vi "Convert_command_string_to_Enum.vi"(5 "Command field in":string, 11 "error in (no error)":errorcluster) -> (6 "mmW_instrument_commands":T1, 10 "Found in Enum?":bool, 15 "error out":errorcluster)   [LabVIEW 2019, in "mmW_commands.lvlib"]
uses:
  mmW_commands.lvlib
  TypeDefs/commands.ctl
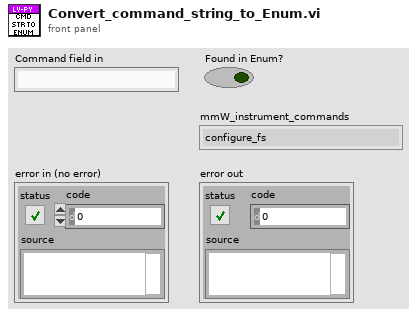
[diagram p1: front panel]
types:
  T1 = typedef "mmW_commands.lvlib/commands.ctl" = enum16{"configure_fs", "configure_rf", "configure_trigger", "equalization_enable", "equalization_start", "lo_sync_enable", "equalization_stop", "get_instrument_status", "get_versions", "initialize_hw", "pop_rx", "set_log_level", "Shutdown", "start", "start_instrument_app", "stop", "transceive", "trigger_burst", "trigger_sync_enable", "Write TX", "resp_generic", "resp_waveform"}
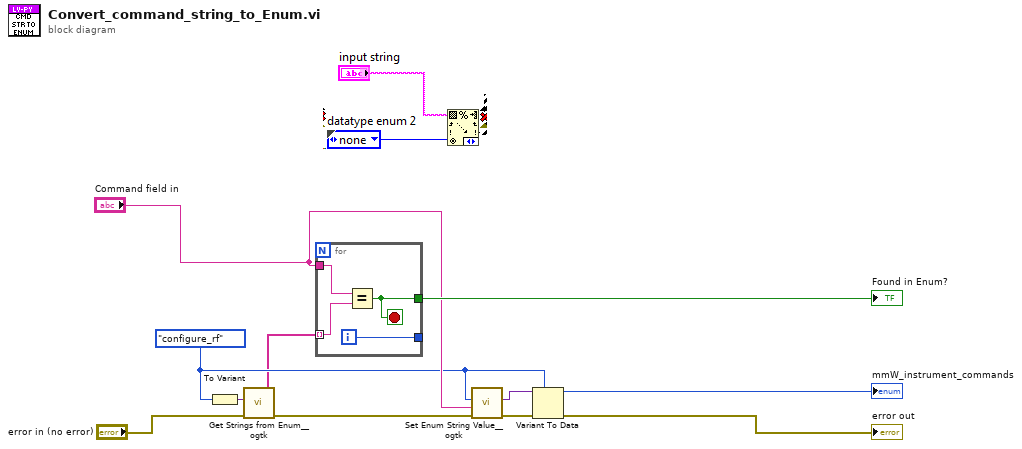
[diagram p0: block diagram]
diagram:
  w5 = commands."configure_rf" ("mmW_instrument_commands")
  n1 = To Variant(anything=w5) -> (Variant=w2:variant)
  n2 = call <userlib>:"Get Strings from Enum__ogtk.vi"("error in (no error)"="error in (no error)", "Enum"=w2) -> ("error out"=w7:errorcluster, "Enum Strings"=w3:string[])  [unwired: 6 in, 2 out]
  n3 = for {
    tunnel: "Command field in" -> [w15]
    tunnel: w3 -> [w14] mode=indexing
    tunnel: [w13] -> w11
    tunnel: [w12] -> _
    i -> [w12]
    stop <- w13 stop-if-true
    n4 = Equal?(x=w15, y=w14) -> (x = y?=w13:bool)
  }
  "Found in Enum?" <- w11
  n5 = call <userlib>:"Set Enum String Value__ogtk.vi"("error in (no error)"=w7, "String Value"="Command field in", "Default Enum Value"=w5) -> ("error out"=w6:errorcluster, "Enum"=w4:variant)  [unwired: 7 in]
  n6 = Variant To Data(error in=w6, type=w5, Variant=w4) -> (data=→"mmW_instrument_commands":T1, error out=→"error out":errorcluster)
